vi "Initialize Value Expressions.vi"(8 "error in (no error)":errorcluster, 10 "Value strings":string[](array[string]), 11 "Output Sequencer in":refnum<class "Output Sequencer.lvclass">) -> (0 "error out":errorcluster, 2 "Expressions":T1[](array[typedef]), 3 "Output Sequencer out":refnum<class "Output Sequencer.lvclass">)   [LabVIEW 2024, in "Output Sequencer.lvlib" / "Output Sequencer.lvclass"]
uses:
  Output Sequencer.lvclass
  Types/Expression Data.ctl
  <vilib>/LAVA/muParser/mupExpr/mupExpr.lvclass
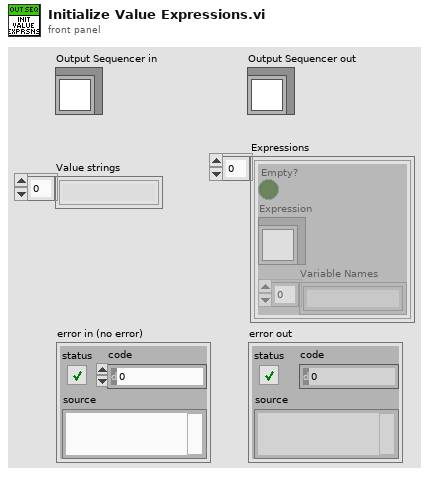
[diagram p1: front panel]
types:
  T1 = typedef "Output Sequencer.lvlib/Output Sequencer.lvclass/Expression Data.ctl" = cluster{"Empty?":bool, "Expression":refnum<class "mupExpr.lvclass">, "Variable Names":string[]}
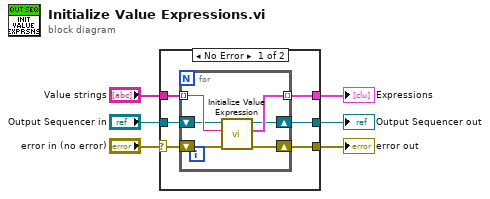
[diagram p0: block diagram]
diagram:
  n1 = case shown="No Error" "error in (no error)" {
    selector: "error in (no error)" -> [w7 w20]
    tunnel: [w12 _] -> w6
    tunnel: "Value strings" -> [w11 _]
    tunnel: "Output Sequencer in" -> [w10 w19]
    tunnel: [w9 w19] -> w3
    tunnel: [w8 w20] -> w2
    frame No Error {
      n2 = for {
        tunnel: w11 -> [w18] mode=indexing
        tunnel: [w17] -> w12 mode=indexing
        shift-right: [w15] -> w9
        shift-left: w10 -> [w16]
        shift-right: [w13] -> w8
        shift-left: w7 -> [w14]
        n3 = call "Initialize Value Expression.vi"("error in (no error)"=w14, "Expression string"=w18, "Output Sequencer in"=w16) -> ("error out"=w13:errorcluster, "Expression Data"=w17:T1, "Output Sequencer out"=w15:refnum<class "Output Sequencer.lvclass">)  [unwired: 6 in]
      }
    }
    frame Error {
    }
  }
  "Expressions" <- w6
  "Output Sequencer out" <- w3
  "error out" <- w2
